vi "Reference Enqueue Message.vi"   [LabVIEW 2021, in "Message Queue.lvlib"]
doc: "For a regular message, enqueue the message. For a priority message, enqueue it at the front of the queue."
uses:
  Message Queue.lvlib
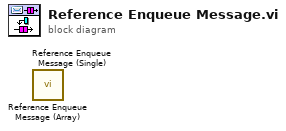
[diagram p0: block diagram]
diagram:
  n1 = call "Reference Enqueue Message (Array).vi"() -> ()  [unwired: 11 in, 1 out]
  n2 = call "Reference Enqueue Message (Single).vi"() -> ()  [unwired: 11 in, 1 out]
